vi "IsCellArrayOfStrings.vi"(11 "ElementType in":refnum<class "ElementType.lvclass">) -> (2 "IsCellArrayOfStrings?":bool, 3 "ElementType out":refnum<class "ElementType.lvclass">)   [LabVIEW 2021]
uses:
  <vilib>/imath/engines/lvmath2/MathScriptCompiler/Type/ElementType.llb/ElementType.lvclass
  <vilib>/imath/engines/lvmath2/MathScriptCompiler/Type/StructEltType.llb/StructEltType.lvclass
  <vilib>/imath/engines/lvmath2/RunTimeEngine/Struct/NIMS_Struct_Global.vi
  <vilib>/imath/engines/lvmath2/MathScriptCompiler/Type.llb/Type.lvclass
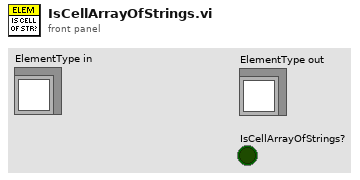
[diagram p1: front panel]
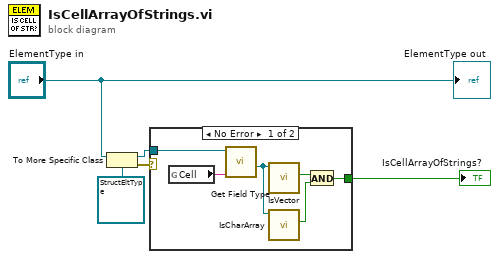
[diagram p0: block diagram]
diagram:
  n1 = To More Specific Class(target class=refnum<class "StructEltType.lvclass"> refnum ("MathScriptTypes.lvlib:StructEltType.lvclass"), reference="ElementType in") -> (specific class reference=w5:refnum<class "StructEltType.lvclass">, error out=w1:errorcluster)  [unwired: 1 in]
  n2 = case shown="No Error" w1 {
    tunnel: w5 -> [w9 _]
    tunnel: [w6 _] -> w2
    frame No Error {
      n3 = global read "NIMS_Struct_Global.vi" "Cell"() -> (w10:string)
      n4 = call <vilib>:"Get Field Type.vi"("Field"=w10, "StructEltType in"=w9) -> ("Data Type"=w11:refnum<class "Type.lvclass">)  [unwired: 5 in, 4 out]
      n5 = call-dynamic "IsVector.vi"("Type in"=w11) -> ("Is Vector?"=w7:bool)  [unwired: 7 in, 3 out]
      n6 = call-dynamic "IsCharArray.vi"("Type in"=w11) -> ("Is Char PlugIn?"=w8:bool)  [unwired: 9 in, 1 out]
      n7 = And(x=w7, y=w8) -> (x .and. y?=w6:bool)
    }
    frame Error {
    }
  }
  "IsCellArrayOfStrings?" <- w2
  "ElementType out" <- "ElementType in"
